vi "Write Menu Button Visible.vi"(5 "Menu Button Visible":bool, 9 "IOName in":refnum<class "IOName.lvclass">) -> (3 "IOName out":refnum<class "IOName.lvclass">)   [LabVIEW 2014, in "Raspberry Pi Compatible Compiler for LabVIEW.lvlib" / "IOName.lvclass"]
uses:
  IOName.lvclass
  IOName.lvclass/IOName.ctl
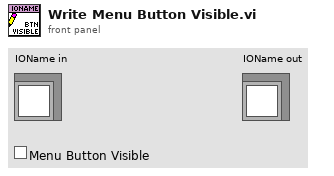
[diagram p1: front panel]
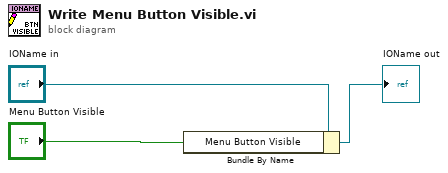
[diagram p0: block diagram]
diagram:
  n1 = Bundle By Name(cluster="IOName in", "Menu Button Visible"="Menu Button Visible") -> (→"IOName out":refnum<class "IOName.lvclass">)
